vi "SRV_Evaluate Sensor Formula.vi"(0 "Sensor Cfg-Command Cluster":T1={"Sensor Config"={"Name"="", "A/D"=enum."Digital", "I2C Address"=0, "Register"=0, "Channel"=0, "Digital Mask"=0, "Units"="", "Sampling Mode"=enum."Polled", "Sample Period (ms)"=1000, "Formula"="", "Sensor View Config"={"Sensor Name"=enum."Gauge 01", "Minimum"=0.0, "Maximum"=10.0}, "Active"=FALSE, "PicoC Shared Var Type"=enum."Integer", "Index"=0, "Stream Multiple?"=FALSE, "Index End"=255, "Bytes"=enum."1 Byte", "Source Sensor Name"="", "Repeat Start"=FALSE, "Integer Word Type"=enum."Unsigned", "Byte Swap"=FALSE}, "Command"="", "Parsed Formula"={"Table"=[], "Y Values"=[]}, "Calculated Sensors Array"=[]} {"Calculated Sensors Array"."Parsed Formula"."Y Values" format="%.2f"; "Calculated Sensors Array"."Sensor Config"."Register" format="%.0x"; "Calculated Sensors Array"."Sensor Config"."I2C Address" format="%.0x"; "Calculated Sensors Array"."Sensor Config"."Sample Period (ms)" min=10 max=60000 step=1; "Calculated Sensors Array"."Sensor Config"."Digital Mask" format="%.0x"; "Calculated Sensors Array"."Sensor Config"."Channel" format="%.0x"; "Parsed Formula"."Y Values" format="%.2f"; "Sensor Config"."Register" format="%.0x"; "Sensor Config"."I2C Address" format="%.0x"; "Sensor Config"."Sample Period (ms)" min=10 max=60000 step=1; "Sensor Config"."Digital Mask" format="%.0x"; "Sensor Config"."Channel" format="%.0x"}, 7 "Value":dbl=nan, 11 "error in (no error)":errorcluster, 12 "Value (U16)":u16, 13 "Value (U8)":u8) -> (8 "Value out":dbl, 15 "error out":errorcluster)   [LabVIEW 2014]
uses:
  SRV_Sensor Config-Command Cluster.ctl
  SRV_Sensor Config Cluster.ctl
  SRV_Sensor Analog-Digital.ctl
  SRV_Sensor Sampling Mode.ctl
  SRV_Sensor View Config Cluster.ctl
  SRV_Sensors Names.ctl
  SRV_Sensor PicoC Shared Var Type.ctl
  SRV_Sensor Number of Bytes.ctl
  SRV_Sensor Integer Word Type.ctl
  SRV_Calculated Sensor Cfg.ctl
  SRV_Sensor Digital Mask Method.ctl
  <vilib>/ptbypt/NI_PtbyPt.lvlib
panel:
  # "operator"
  # "register1"
  # "register2"
  # "operator"
  # "register1"
  # "register2"
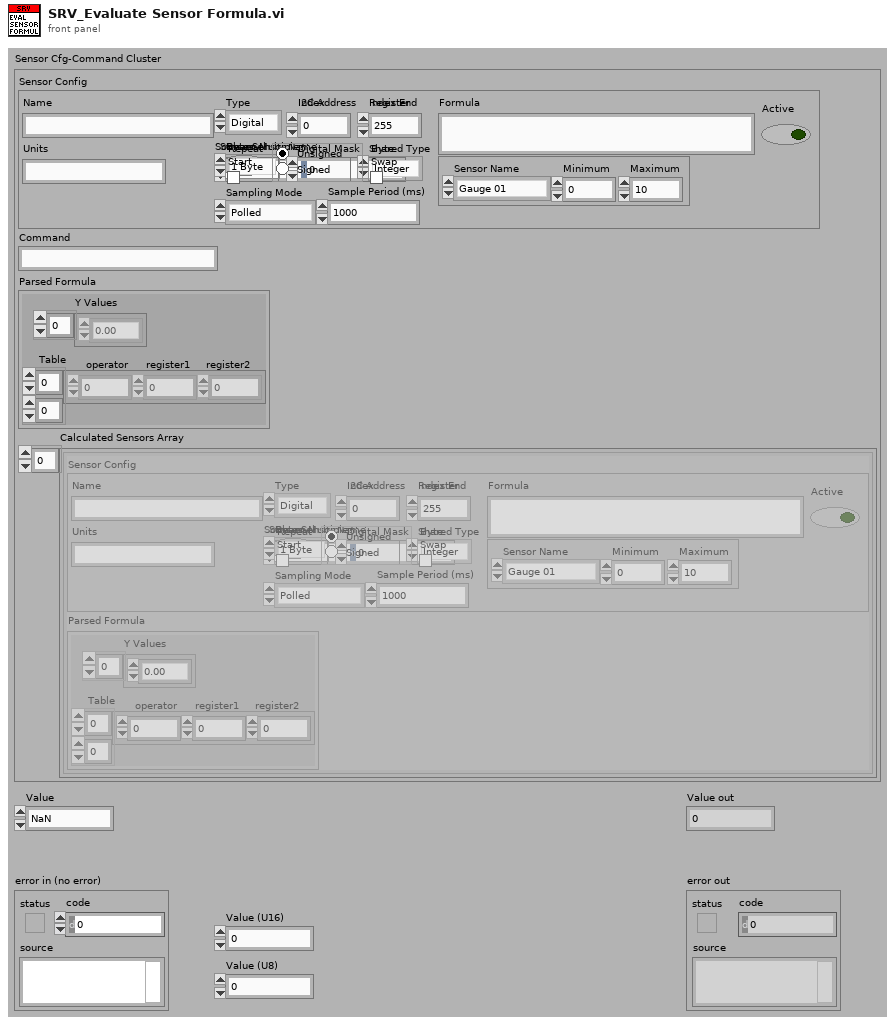
[diagram p1: front panel]
types:
  T1 = typedef "SRV_Sensor Config-Command Cluster.ctl" = cluster{"Sensor Config":T2, "Command":string, "Parsed Formula":cluster{"Table":i32[][], "Y Values":dbl[]}, "Calculated Sensors Array":T10[]}
  T2 = typedef "SRV_Sensor Config Cluster.ctl" = cluster{"Name":string, "A/D":T3, "I2C Address":u8, "Register":u8, "Channel":u8, "Digital Mask":u16, "Units":string, "Sampling Mode":T4, "Sample Period (ms)":u32, "Formula":string, "Sensor View Config":T5, "Active":bool, "PicoC Shared Var Type":T7, "Index":u8, "Stream Multiple?":bool, "Index End":u8, "Bytes":T8, "Source Sensor Name":string, "Repeat Start":bool, "Integer Word Type":T9, "Byte Swap":bool}
  T3 = typedef "SRV_Sensor Analog-Digital.ctl" = enum16{"Digital", "Analog", "PicoC Shared", "Calculated"}
  T4 = typedef "SRV_Sensor Sampling Mode.ctl" = enum16{"Polled", "Streaming"}
  T5 = typedef "SRV_Sensor View Config Cluster.ctl" = cluster{"Sensor Name":T6, "Minimum":dbl, "Maximum":dbl}
  T6 = typedef "SRV_Sensors Names.ctl" = enum16{"Gauge 01", "Gauge 02", "Gauge 03", "Gauge 04", "Meter 01", "Meter 02", "Meter 03", "Meter 04", "Numeric 01", "Numeric 02", "Numeric 03", "Numeric 04", "Numeric 05", "Numeric 06", "Numeric 07", "Numeric 08", "Boolean 01", "Boolean 02", "Boolean 03", "Boolean 04", "Boolean 05", "Boolean 06", "Boolean 07", "Boolean 08", "Boolean 09", "Boolean 10", "Boolean 11", "Boolean 12", "Boolean 13", "Boolean 14", "Boolean 15", "Boolean 16", "Boolean 17", "Boolean 18", "Boolean 19", "Boolean 20", "Boolean 21", "Boolean 22", "Boolean 23", "Boolean 24", "Boolean 25", "Boolean 26", "Boolean 27", "Boolean 28", "Boolean 29", "Boolean 30", "Boolean 31", "Boolean 32"}
  T7 = typedef "SRV_Sensor PicoC Shared Var Type.ctl" = enum16{"String", "Integer", "Float"}
  T8 = typedef "SRV_Sensor Number of Bytes.ctl" = enum16{"1 Byte", "2 Bytes"}
  T9 = typedef "SRV_Sensor Integer Word Type.ctl" = enum32{"Unsigned", "Signed"}
  T10 = typedef "SRV_Calculated Sensor Cfg.ctl" = cluster{"Sensor Config":T2, "Parsed Formula":cluster{"Table":i32[][], "Y Values":dbl[]}}
  T11 = typedef "SRV_Sensor Digital Mask Method.ctl" = enum16{"AND", "OR"}
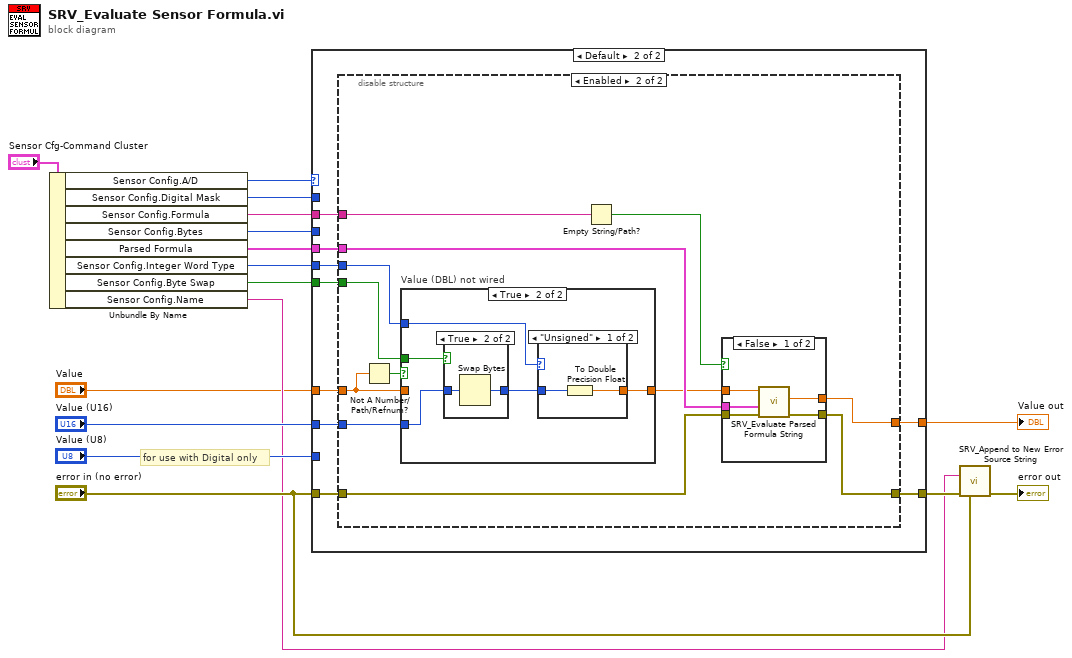
[diagram p0: block diagram]
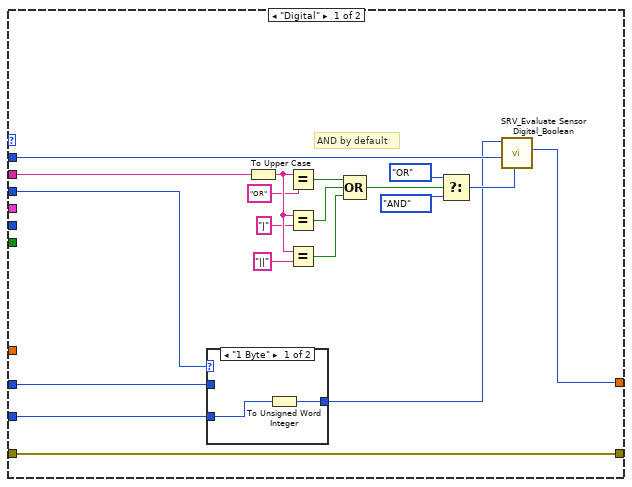
[diagram p2: hidden frame]
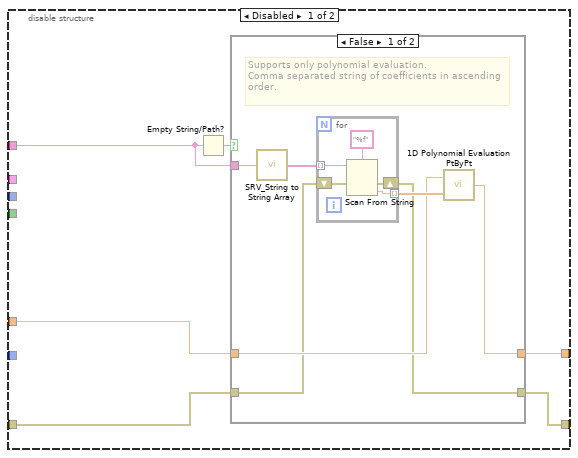
[diagram p4: hidden frame]
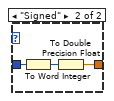
[diagram p8: hidden frame]
diagram:
  # "for use with Digital only"
  n1 = Unbundle By Name("Sensor Cfg-Command Cluster") -> ("Sensor Config.A/D"=w10:T3, "Sensor Config.Digital Mask"=w9:u16, "Sensor Config.Formula"=w15:string, "Sensor Config.Bytes"=w6:T8, "Parsed Formula"=w5:cluster{"Table":i32[][], "Y Values":dbl[]}, "Sensor Config.Integer Word Type"=w4:T9, "Sensor Config.Byte Swap"=w2:bool, "Sensor Config.Name"=w3:string)
  n2 = case shown="Default" w10 {
    tunnel: w15 -> [w17 w47]
    tunnel: "Value" -> [_ w46]
    tunnel: [w23 w45] -> w14
    tunnel: [w22 w44] -> w13
    tunnel: "error in (no error)" -> [w22 w43]
    tunnel: w9 -> [w24 _]
    tunnel: "Value (U16)" -> [w19 w39]
    tunnel: "Value (U8)" -> [w20 _]
    tunnel: w6 -> [w21 _]
    tunnel: w5 -> [_ w42]
    tunnel: w4 -> [_ w41]
    tunnel: w2 -> [_ w40]
    frame "Digital" {
      # "AND by default"
      n3 = case shown="\"1 Byte\"" w21 {
        tunnel: w20 -> [w37 _]
        tunnel: w19 -> [_ w38]
        tunnel: [w36 w38] -> w18
        frame "1 Byte" {
          n4 = To Unsigned Word Integer(number=w37) -> (unsigned 16bit integer=w36:u16)
        }
        frame "2 Bytes" {
        }
      }
      n5 = To Upper Case(1:w17) -> (0:w31:string)
      n6 = Equal?(x=w31, y="OR") -> (x = y?=w28:bool)
      n7 = Equal?(x=w31, y="|") -> (x = y?=w29:bool)
      n8 = Equal?(x=w31, y="||") -> (x = y?=w30:bool)
      n9 = Compound Arithmetic op=OR(w28, w29, w30) -> (w32:bool)
      n10 = Select(t=SRV_Sensor_Digital_Mask_Method."OR" ("Mask Method (AND)"), s=w32, f=SRV_Sensor_Digital_Mask_Method."AND" ("Mask Method (AND)")) -> (s? t:f=w34:T11)
      n11 = call "SRV_Evaluate Sensor Digital_Boolean.vi"("Mask Method (AND)"=w34, "Mask"=w24, "Value (U16)"=w18) -> ("Result"=w23:u8)  [unwired: 7 in, 1 out]
    }
    frame Default {
      n12 = disable-structure shown="Enabled" {
        disable-tunnel: w47 -> [w48 w75]
        disable-tunnel: w46 -> [w53 w69]
        disable-tunnel: [w51 w76] -> w45
        disable-tunnel: [w50 w77] -> w44
        disable-tunnel: w43 -> [w49 w78]
        disable-tunnel: w42 -> [_ w79]
        disable-tunnel: w41 -> [_ w73]
        disable-tunnel: w40 -> [_ w71]
        disable-tunnel: w39 -> [_ w70]
        frame Disabled {
          n13 = Empty String/Path?(string/path=w48) -> (empty?=w52:bool)
          n14 = case shown="False" w52 {
            tunnel: w53 -> [w57 w66]
            tunnel: [w56 w66] -> w51
            tunnel: w48 -> [w60 _]
            tunnel: [w54 w67] -> w50
            tunnel: w49 -> [w55 w67]
            frame False {
              # "Supports only polynomial evaluation.\nComma separated string of coefficients in ascending order."
              n15 = call "SRV_String to String Array.vi"("String"=w60) -> ("String Array"=w59:string[])  [unwired: 14 in]
              n16 = for {
                tunnel: [w63] -> w58 mode=indexing
                tunnel: w59 -> [w65] mode=indexing
                shift-right: [w61] -> w54
                shift-left: w55 -> [w62]
                n17 = Scan From String(format string="%f", input string=w65, error in=w62) -> (error out=w61:errorcluster, output 1=w63:dbl)  [unwired: 2 in, 2 out]
              }
              n18 = call <vilib>:"1D Polynomial Evaluation PtByPt.vi"("Coefficients: a"=w58, "x"=w57) -> ("y"=w56:dbl)
            }
            frame True {
            }
          }
        }
        frame Enabled {
          n19 = Not A Number/Path/Refnum?(number/path/refnum=w69) -> (NaN/Path/Refnum?=w68:bool)
          n20 = case "Value (DBL) not wired" shown="True" w68 {
            tunnel: w73 -> [_ w85]
            tunnel: [w80 w81] -> w72
            tunnel: w69 -> [w80 _]
            tunnel: w71 -> [_ w83]
            tunnel: w70 -> [_ w82]
            frame False {
              # "Value DBL is wired\n(e.g. Pico C)"
            }
            frame True {
              n21 = case shown="True" w83 {
                tunnel: w82 -> [w86 w88]
                tunnel: [w86 w87] -> w84
                frame False {
                }
                frame True {
                  n22 = Swap Bytes(anything=w88) -> (byte swapped=w87:u16)
                }
              }
              n23 = case shown="\"Unsigned\"" w85 {
                tunnel: w84 -> [w90 w92]
                tunnel: [w89 w91] -> w81
                frame "Unsigned" {
                  n24 = To Double Precision Float(number=w90) -> (double precision float=w89:dbl)
                }
                frame "Signed" {
                  n25 = To Word Integer(number=w92) -> (16bit integer=w93:i16)
                  n26 = To Double Precision Float(number=w93) -> (double precision float=w91:dbl)
                }
              }
            }
          }
          n27 = Empty String/Path?(string/path=w75) -> (empty?=w74:bool)
          n28 = case shown="False" w74 {
            tunnel: w79 -> [w98 _]
            tunnel: w78 -> [w97 w99]
            tunnel: [w96 w99] -> w77
            tunnel: [w95 w100] -> w76
            tunnel: w72 -> [w94 w100]
            frame False {
              n29 = call "SRV_Evaluate Parsed Formula String.vi"("error in (no error)"=w97, "Parsed Formula"=w98, "Variable v"=w94) -> ("error out"=w96:errorcluster, "Value out"=w95:dbl)  [unwired: 7 in]
            }
            frame True {
            }
          }
        }
      }
    }
  }
  "Value out" <- w14
  n30 = call "SRV_Append to New Error Source String.vi"("Message String to append"=w3, "Error In (no error)"=w13, "Previous Error In (no error)"="error in (no error)") -> ("error out"=→"error out":errorcluster)  [unwired: 12 in]
